vi "Set Multi Gate Peaks In Gate [PMG].vi"(6 "Gate Number":i32, 7 "Micropulse # In":i32, 8 "error in (no error)":errorcluster, 9 "# Peaks In Gate":u16, 11 "Test Number":u32) -> (0 "error out":errorcluster, 5 "Micropulse # Out":i32)   [LabVIEW 2026, in "MicroPulse_Driver.lvlib"]
doc: "Multi-gate version of PIG command Used to define how many peaks are reported in AMM mode 2. The first n-1 plus the largest of the remaining peaks are reported.\n\nParameters:\n<Tn> : Test number. An integer value from 0 to the maximum number of tests (default maximum is 1279 tests).\nTn = 0 for all conventional tests. If the S extension is used it applies to all tests in the sweep number specified: 1-32, 0 = all sweeps\n\n<Gn> : Gate Number, an integer value from 0 to 4.\nGn = 0 for all gates in the test\n\n<Value> : Integer value n from 1 to 80\n\nNote: Valid in Multi-gate Mode only (AMP 31 & 32)"
uses:
  MicroPulse_Driver.lvlib
  Private/MP-Registry Action-Enum.ctl
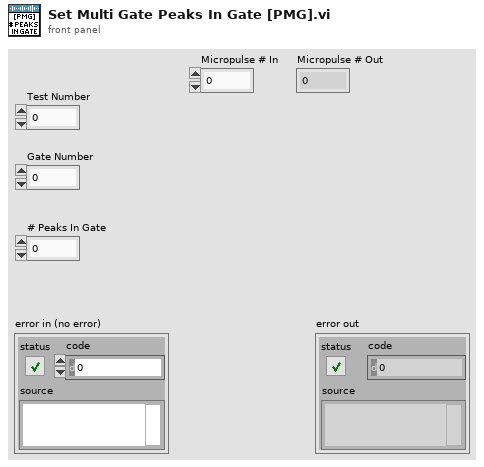
[diagram p1: front panel]
types:
  T1 = typedef "MicroPulse_Driver.lvlib/MP-Registry Action-Enum.ctl" = enum16{"Read", "Add Test", "Add Command", "Add Gate Command", "Add Encoder Command", "Clear Command  List", "Set Registry", "Set System Details", "Set DOF", "Set Velocity", "Disable Asynch Reads", "Enable Asynch Reads", "Add Connection", "Disconnect", "Shutdown"}
  T2 = typedef "Micropulse.lvlib/TCP config.ctl" = cluster{"Connection ID":refnum<k5>, "IP address":string, "host port":u16, "OC timeout":i32, "Read timeout":i32, "Write timeout":i32}
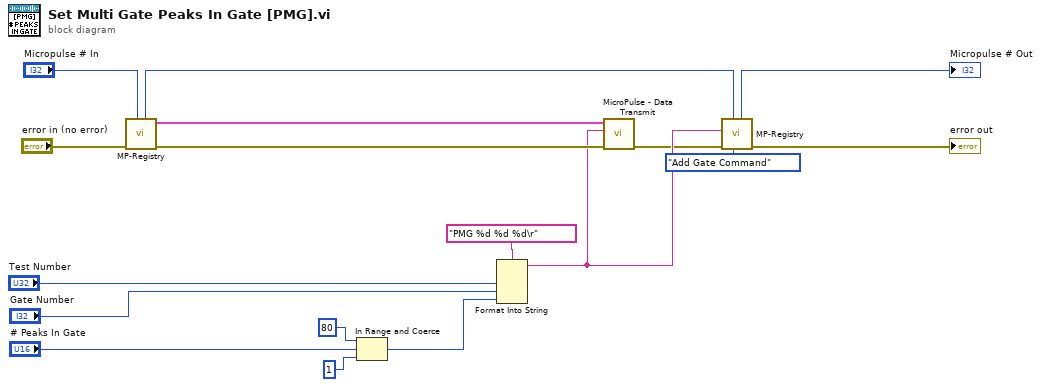
[diagram p0: block diagram]
diagram:
  n1 = call "MP-Registry.vi"("Micropulse # In"="Micropulse # In", "error in (no error)"="error in (no error)") -> ("error out"=w15:errorcluster, "TCP config"=w14:T2, "Micropulse # Out"=w8:i32)  [unwired: 6 in, 1 out]
  n2 = In Range and Coerce(upper limit=u16 80, x="# Peaks In Gate", lower limit=u16 1) -> (coerced(x)=w3:u16)  [unwired: 1 out]
  n3 = Format Into String(format string="PMG %d %d %d\r", "Test Number", "Gate Number", w3) -> (resulting string=w12:string)  [unwired: 2 in, 1 out]
  n4 = call "MicroPulse - Data Transmit.vi"("error in (no error)"=w15, "data"=w12, "TCP config"=w14) -> ("error out"=w10:errorcluster)  [unwired: 6 in, 2 out]
  n5 = call "MP-Registry.vi"("Action"=MP-Registry_Action-Enum."Add Gate Command", "Micropulse # In"=w8, "error in (no error)"=w10, "Data in"=w12) -> ("error out"=→"error out":errorcluster, "Micropulse # Out"=→"Micropulse # Out":i32)  [unwired: 4 in, 2 out]
